vi "FindClosestTarget.vi"(10 "Find Y? (F)":bool, 11 "Targets To Sort":T1(array[cluster])) -> (1 "Index":dbl, 2 "Distance (ft)":dbl, 3 "Target Center (-1 to 1)":cluster{"X":dbl, "Y":dbl})   [LabVIEW 2011]
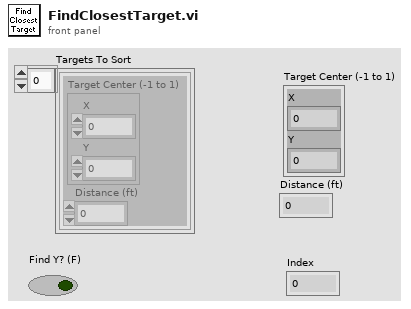
[diagram p1: front panel]
types:
  T1 = cluster{"Target Center (-1 to 1)":cluster{"X":dbl, "Y":dbl}, "Distance (ft)":dbl}[]
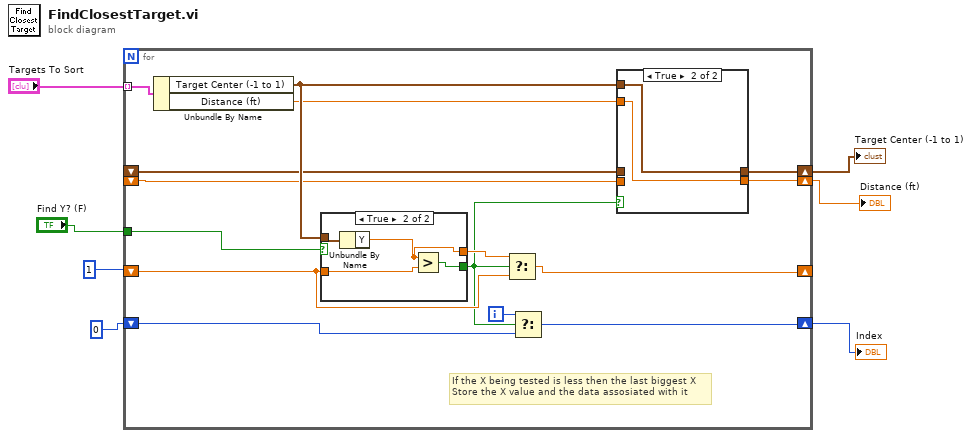
[diagram p0: block diagram]
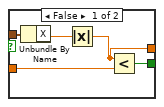
[diagram p2: hidden frame]
diagram:
  n1 = for {
    tunnel: "Targets To Sort" -> [w22] mode=indexing
    shift-right: [w18] -> w4
    shift-left: _ -> [w16]
    shift-right: [w19] -> w5
    shift-left: _ -> [w17]
    shift-right: [w14] -> _
    shift-left: 1 -> [w15]
    tunnel: "Find Y? (F)" -> [w8]
    shift-right: [w12] -> w2
    shift-left: 0 -> [w9]
    i -> [w10]
    # "If the X being tested is less then the last biggest X\nStore the X value and the data assosiated with it"
    n2 = Unbundle By Name(w22) -> ("Target Center (-1 to 1)"=w21:cluster{"X":dbl, "Y":dbl}, "Distance (ft)"=w20:dbl)
    n3 = case shown="True" w8 {
      tunnel: w21 -> [w27 w31]
      tunnel: w15 -> [w26 w29]
      tunnel: [w24 w28] -> w13
      tunnel: [w23 w30] -> w11
      frame False {
        n4 = Unbundle By Name(w27) -> ("X"=w25:dbl)
        n5 = Absolute Value(x=w25) -> (abs(x)=w24:dbl)
        n6 = Less?(x=w24, y=w26) -> (x < y?=w23:bool)
      }
      frame True {
        n7 = Unbundle By Name(w31) -> ("Y"=w28:dbl)
        n8 = Greater?(x=w28, y=w29) -> (0:w30:bool)
      }
    }
    n9 = Select(t=w13, s=w11, f=w15) -> (s? t:f=w14:dbl)
    n10 = Select(t=w10, s=w11, f=w9) -> (s? t:f=w12:i32)
    n11 = case shown="True" w11 {
      tunnel: w21 -> [_ w34]
      tunnel: w20 -> [_ w35]
      tunnel: [w32 w35] -> w18
      tunnel: [w33 w34] -> w19
      tunnel: w17 -> [w33 _]
      tunnel: w16 -> [w32 _]
      frame False {
      }
      frame True {
      }
    }
  }
  "Distance (ft)" <- w4
  "Target Center (-1 to 1)" <- w5
  "Index" <- w2
